vi "SwitchPacketParser.vi"(4 "Message":u8[](array[numeric])) -> (1 "switch Packet Out":T1)   [LabVIEW 2014]
uses:
  switchPacket.ctl
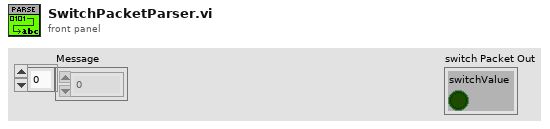
[diagram p1: front panel]
types:
  T1 = typedef "switchPacket.ctl" = cluster{"switchValue":bool}
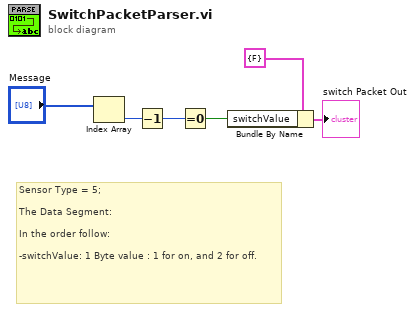
[diagram p0: block diagram]
diagram:
  # "Sensor Type = 5;\n\nThe Data Segment:\n\nIn the order follow:\n\n-switchValue: 1 Byte value : 1 for on, and 2 for off."
  n1 = Index Array(array="Message") -> (element=w5:u8)  [unwired: 1 in]
  n2 = Decrement(x=w5) -> (x-1=w4:u8)
  n3 = Equal To 0?(x=w4) -> (x = 0?=w3:bool)
  n4 = Bundle By Name(cluster=T1 {"switchValue"=FALSE} ("switchPacket"), "switchValue"=w3) -> (→"switch Packet Out":T1)
